vi "Coordinates Overlapping.vi"(10 "Tail Positions":T1, 11 "Head Position":T1) -> (3 "Checkbox":bool)   [LabVIEW 2021]
uses:
  Positions.ctl
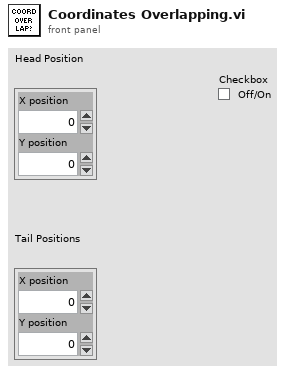
[diagram p1: front panel]
types:
  T1 = typedef "Positions.ctl" = cluster{"X position":i32, "Y position":i32}
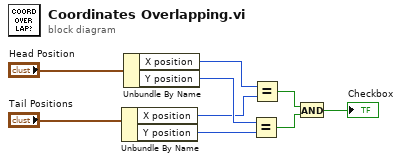
[diagram p0: block diagram]
diagram:
  n1 = Unbundle By Name("Tail Positions") -> ("X position"=w4:i32, "Y position"=w6:i32)
  n2 = Unbundle By Name("Head Position") -> ("X position"=w3:i32, "Y position"=w5:i32)
  n3 = Equal?(x=w5, y=w6) -> (x = y?=w7:bool)
  n4 = Equal?(x=w3, y=w4) -> (x = y?=w8:bool)
  n5 = And(x=w8, y=w7) -> (x .and. y?=→"Checkbox":bool)
